vi "fpga_Previous Integration (DT Reset).vi"(6 "instantaneous reset after tripping? (F)":bool, 7 "integrate?":bool, 8 "input valid":bool=TRUE, 9 "start signal? (F)":bool, 10 "channel index":u8, 11 "dt/T":fxp<+/-,32,1>) -> (0 "output valid":bool, 2 "integrated value":fxp<+,32,0>, 3 "trip?":bool)   [LabVIEW 2012, in "NI_EP_Protection_FPGA.lvlib"]
uses:
  <vilib>/addons/Electrical Power/Protection/NI_EP_Protection_FPGA.lvlib
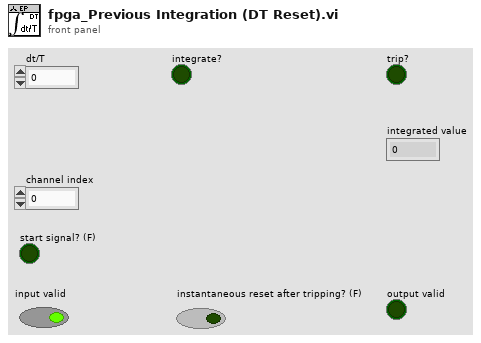
[diagram p1: front panel]
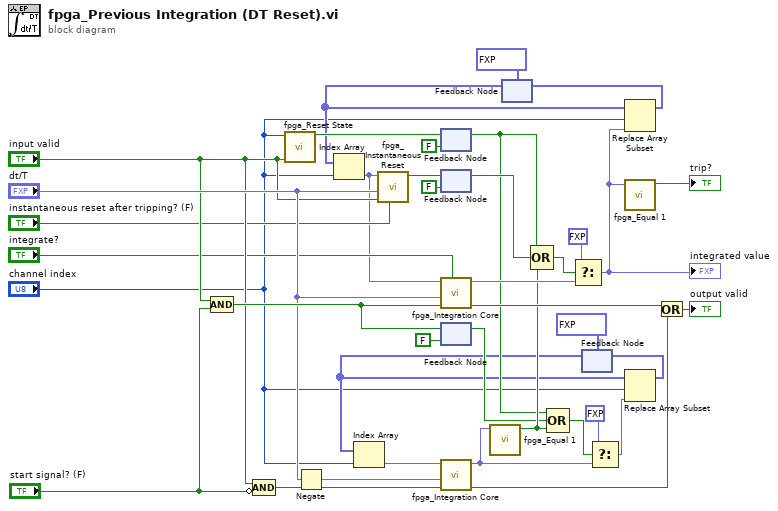
[diagram p0: block diagram]
diagram:
  n1 = Compound Arithmetic op=AND("input valid", "start signal? (F)") -> (w22:bool)
  n2 = Compound Arithmetic op=AND("input valid", invert "start signal? (F)") -> (w25:bool)
  n3 = call <vilib>:"fpga_Reset State.vi"("input valid"="input valid", "channel index"="channel index") -> ("reset?"=w6:bool)  [unwired: 9 in]
  n4 = Negate(x="dt/T") -> (-x=w24:fxp<+/-,32,1>)
  n5 = feedback #1(FALSE) -> (w7:bool)
  n6 = feedback-in #1(w6) -> ()
  n7 = feedback #2(FALSE) -> (w19:bool)
  n8 = feedback #3(FALSE) -> (w8:bool)
  n9 = feedback-in #3(w22) -> ()
  n10 = feedback #4(fxp<+,32,0>[] [0.0, 0.0, 0.0, 0.0, 0.0, 0.0, 0.0, 0.0, 0.0, 0.0, 0.0, 0.0, 0.0, 0.0, 0.0, 0.0]) -> (w5:fxp<+,32,0>[])
  n11 = Index Array(array=w5, index="channel index") -> (element=w4:fxp<+,32,0>)
  n12 = call <vilib>:"fpga_Instantaneous Reset.vi"("instantaneous reset after tripping? (F)"="instantaneous reset after tripping? (F)", "input valid"="input valid", "dt/T"="dt/T", "previous integrated value"=w4) -> ("instantaneous reset?"=w17:bool)  [unwired: 7 in]
  n13 = feedback-in #2(w17) -> ()
  n14 = call <vilib>:"fpga_Integration Core.vi"("integrate?"="integrate?", "input valid"=w22, "dt/T"="dt/T", "previous integrated value"=w4) -> ("output valid"=w21:bool, "integrated value out"=w20:fxp<+,32,0>)  [unwired: 6 in]
  n15 = feedback #5(fxp<+,32,0>[] [0.0, 0.0, 0.0, 0.0, 0.0, 0.0, 0.0, 0.0, 0.0, 0.0, 0.0, 0.0, 0.0, 0.0, 0.0, 0.0]) -> (w3:fxp<+,32,0>[])
  n16 = Index Array(array=w3, index="channel index") -> (element=w1:fxp<+,32,0>)
  n17 = call <vilib>:"fpga_Integration Core.vi"("input valid"=w25, "dt/T"=w24, "previous integrated value"=w1) -> ("output valid"=w23:bool, "integrated value out"=w13:fxp<+,32,0>)  [unwired: 7 in]
  n18 = call <vilib>:"fpga_Equal 1.vi"("data in 32.0"=w13) -> ("=1?"=w12:bool)  [unwired: 10 in]
  n19 = Compound Arithmetic op=OR(w7, w19, w12) -> (w36:bool)
  n20 = Compound Arithmetic op=OR(w7, w8, w12) -> (w30:bool)
  n21 = Select(t=fxp<+,32,0> 0.0 ("f"), s=w36, f=w20) -> (s? t:f=w15:fxp<+,32,0>)
  "integrated value" <- w15
  n22 = Select(t=fxp<+,32,0> 0.0 ("f"), s=w30, f=w13) -> (s? t:f=w34:fxp<+,32,0>)
  n23 = Replace Array Subset(array=w5, new element=w15, index="channel index") -> (w37:fxp<+,32,0>[])
  n24 = feedback-in #4(w37) -> ()
  n25 = call <vilib>:"fpga_Equal 1.vi"("data in 32.0"=w15) -> ("=1?"=→"trip?":bool)  [unwired: 10 in]
  n26 = Replace Array Subset(array=w3, new element=w34, index="channel index") -> (w33:fxp<+,32,0>[])
  n27 = feedback-in #5(w33) -> ()
  n28 = Or(x=w21, y=w23) -> (x .or. y?=→"output valid":bool)
